vi "LabJackT7I2C.vi"(4 "Scan Period":dbl format="%.2f", 5 "Previous Scan Value":dbl format="%.2f", 6 "Present scan array":dbl[](array[numeric]) format="%.2f", 7 "Value to Output":dbl format="%.2f", 8 "Ch Description":T1={"Ch Name"="", "Type"="", "Function"=enum."Analogue Input", "Ch State"=enum."On", "Calibration type"=enum."Raw", "A"=2.0, "B"=3.0, "C"=224.0, "D"=5.0, "Comments"="", "Address"={"Main"=502, "Ch."=0, "Sub"=0, "Port Name"="192.168.124.53"}, "String"="", "Duty"=65535} {"Duty" format="%.0b"; "D" format="%#_5g"; "C" format="%#_5g"; "B" format="%#_5g"; "A" format="%#_5g"}, 9 "Ch names":string[](array[string])) -> (0 "Scan comment":string, 1 "Output":dbl=101.0 format="%.7f")   [LabVIEW 2015]
uses:
  ADAM Client/Sub VIs/ADAM Controls/Ch_description_ADAM.ctl
  ADAM Client/Sub VIs/ADAM Controls/Module_type_ADAM.ctl
  ADAM Client/Sub VIs/ADAM Controls/Function_ADAM.ctl
  ADAM Client/Sub VIs/ADAM Controls/Channel_State.ctl
  ADAM Client/Sub VIs/ADAM Controls/Calib_type_ADAM.ctl
  ADAM Client/Sub VIs/ADAM Controls/Address.ctl
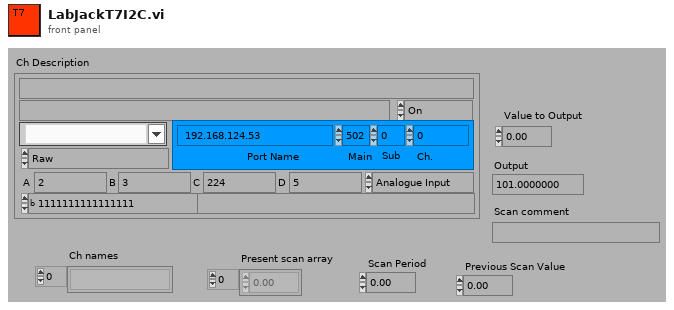
[diagram p1: front panel]
types:
  T1 = typedef "Ch_description_ADAM.ctl" = cluster{"Ch Name":string, "Type":T2, "Function":T3, "Ch State":T4, "Calibration type":T5, "A":dbl, "B":dbl, "C":dbl, "D":dbl, "Comments":string, "Address":T6, "String":string, "Duty":u16}
  T2 = typedef "Module_type_ADAM.ctl" = string
  T3 = typedef "Function_ADAM.ctl" = enum16{"Analogue Input", "Digital Input", "Event counter", "Event rate", "Analogue Output", "Digital Output", "Relay Output"}
  T4 = typedef "Channel_State.ctl" = enum16{"On", "Off", "Always On", "Always Off"}
  T5 = typedef "Calib_type_ADAM.ctl" = enum16{"Raw", "Bx + A", "Cx^2 + Bx + A", "Dx^3 + Cx^2 + Bx + A", "In Band", "Hi-Tec Q", "Hi-Tec M_dot", "Text"}
  T6 = typedef "Address.ctl" = cluster{"Main":i32, "Ch.":i32, "Sub":i32, "Port Name":string}
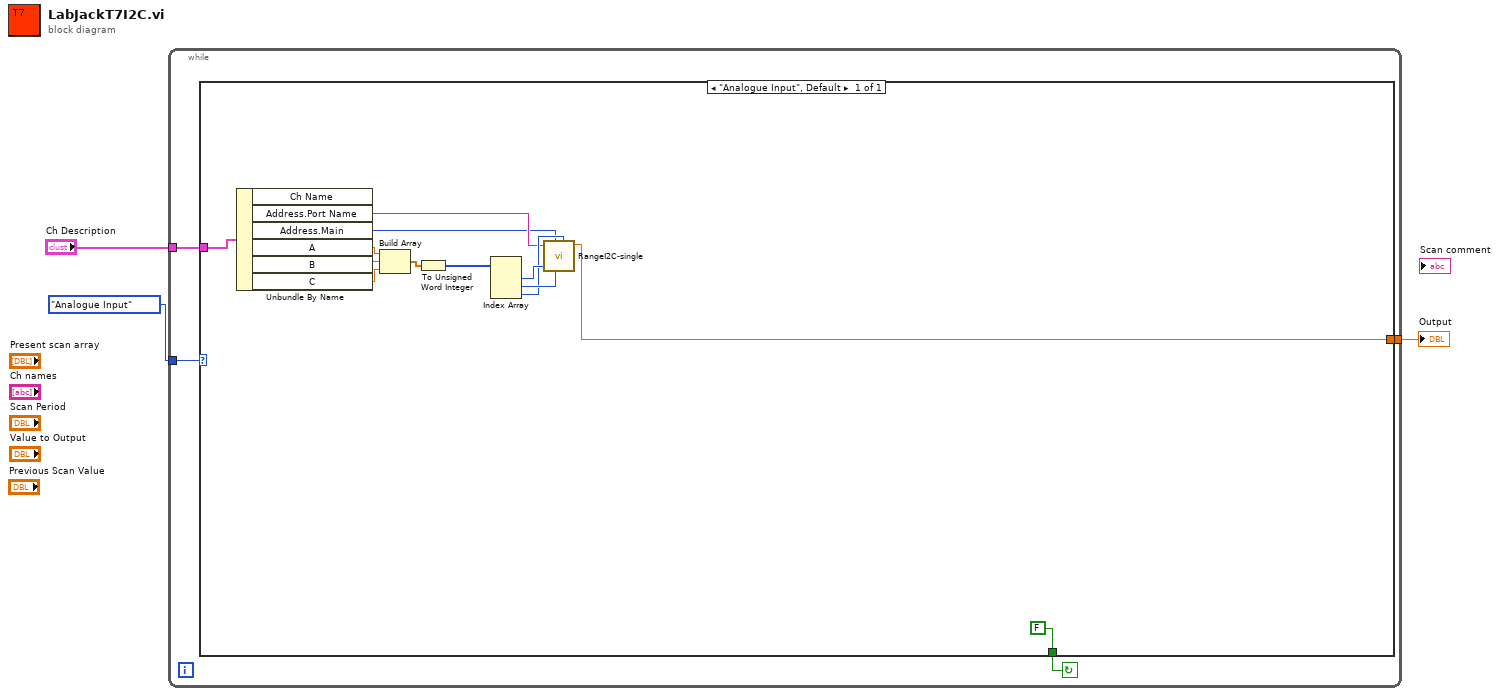
[diagram p0: block diagram]
diagram:
  n1 = while {
    tunnel: "Ch Description" -> [w7]
    tunnel: [w6] -> w2
    tunnel: Function_ADAM."Analogue Input" ("Function") -> [w5]
    stop <- w4 continue-if-true
    n2 = case shown="\"Analogue Input\", Default" w5 {
      tunnel: w7 -> [w20]
      tunnel: [w12] -> w6
      tunnel: [FALSE] -> w4
      frame "Analogue Input", Default {
        n3 = Unbundle By Name(w20) -> ("Address.Port Name"=w14:string, "Address.Main"=w13:i32, "A"=w10:dbl, "B"=w9:dbl, "C"=w8:dbl)  [unwired: 1 out]
        n4 = Build Array(w10, w9, w8) -> (w19:dbl[])
        n5 = To Unsigned Word Integer(number=w19) -> (unsigned 16bit integer=w18:u16[])
        n6 = Index Array(array=w18) -> (element #1=w17:u16, element #2=w16:u16, element #3=w15:u16)  [unwired: 3 in]
        n7 = call "RangeI2C-single.vi"("Remote IP Address"=w14, "Remote Port"=w13, "SCL DIO Ch. No."=w17, "SDA DIO Ch. No."=w16, "CURRENT 8-bit address (dec.)"=w15) -> ("Range (cm)"=w12:dbl)  [unwired: 4 in, 1 out]
      }
    }
  }
  "Output" <- w2
